vi "GET_2D_Histo_bins_(all_types).vi"   [LabVIEW 2018, in "Tracker.lvlib"]
uses:
  Tracker.lvlib
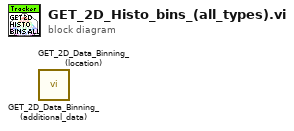
[diagram p0: block diagram]
diagram:
  n1 = call "GET_2D_Data_Binning_(additional_data).vi"() -> ()  [unwired: 5 in, 1 out]
  n2 = call "GET_2D_Data_Binning_(location).vi"() -> ()  [unwired: 5 in, 1 out]
